vi "计算线段的垂直平分线.vi"(8 "Error In":errorcluster caption="错误输入", 11 "线段":T1) -> (0 "Error Out":errorcluster caption="错误输出", 3 "斜率与截距":T3)   [LabVIEW 2012, in "几何工具.lvlib"]
uses:
  <vilib>/Utility/miscctls.llb/LVPointDoubleTypeDef.ctl
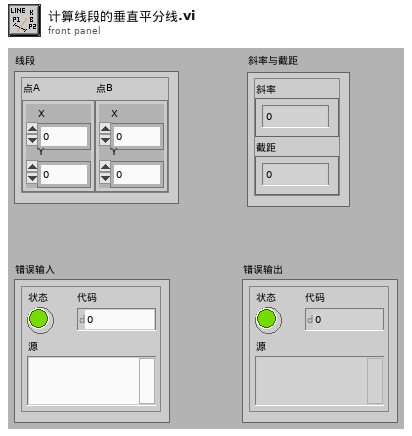
[diagram p1: front panel]
types:
  T1 = typedef "两点直线.ctl" = cluster{"点A":T2, "点B":T2}
  T2 = typedef "LVPointDoubleTypeDef.ctl" = cluster{"X":dbl, "Y":dbl}
  T3 = typedef "几何工具.lvlib/斜率与截距.ctl" = cluster{"斜率":dbl, "截距":dbl}
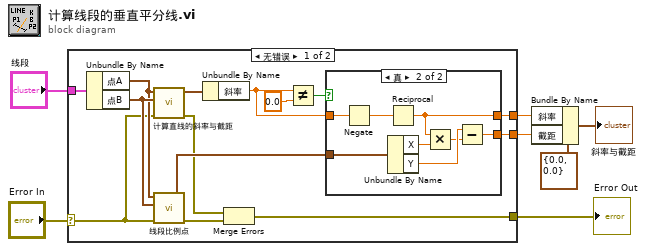
[diagram p0: block diagram]
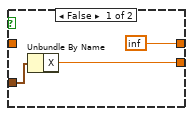
[diagram p2: hidden frame]
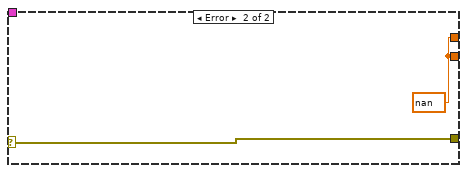
[diagram p3: hidden frame]
diagram:
  n1 = case shown="无错误" "Error In" {
    selector: "Error In" -> [w12 w34]
    tunnel: "线段" -> [w21 _]
    tunnel: [w17 w33] -> w5
    tunnel: [w16 w33] -> w4
    tunnel: [w9 w34] -> w1
    frame No Error {
      n2 = Unbundle By Name(w21) -> ("点A"=w15:T2, "点B"=w20:T2)
      n3 = call "计算直线的斜率与截距.vi"("Error In"=w12, "点B"=w20, "点A"=w15) -> ("Error Out"=w11:errorcluster, "斜率与截距"=w18:T3)  [unwired: 7 in]
      n4 = call "线段比例点.vi"("Error In"=w12, "点B"=w20, "点A"=w15) -> ("Error Out"=w10:errorcluster, "比例点"=w19:T2)  [unwired: 7 in]
      n5 = Unbundle By Name(w18) -> ("斜率"=w13:dbl)
      n6 = Merge Errors(w11, w10) -> (w9:errorcluster)
      n7 = Not Equal?(x=w13, y=0.0) -> (x != y?=w14:bool)
      n8 = case shown="真" w14 {
        tunnel: w19 -> [w24 w32]
        tunnel: w13 -> [_ w27]
        tunnel: [inf w26] -> w17
        tunnel: [w23 w25] -> w16
        frame False {
          n9 = Unbundle By Name(w24) -> ("X"=w23:dbl)
        }
        frame True {
          n10 = Negate(x=w27) -> (-x=w28:dbl)
          n11 = Reciprocal(x=w28) -> (1/x=w26:dbl)
          n12 = Unbundle By Name(w32) -> ("X"=w31:dbl, "Y"=w30:dbl)
          n13 = Multiply(x=w26, y=w31) -> (x*y=w29:dbl)
          n14 = Subtract(x=w30, y=w29) -> (x-y=w25:dbl)
        }
      }
    }
    frame Error {
      w33 = nan ("斜率")
    }
  }
  "Error Out" <- w1
  n15 = Bundle By Name(cluster=T3 {"斜率"=0.0, "截距"=0.0} ("斜率与截距"), "斜率"=w5, "截距"=w4) -> (→"斜率与截距":T3)
